vi "GetGrabberPositions.vi"(0 "reference":refnum<class "PackageNode.lvclass">, 5 "error in (no error)":errorcluster) -> (14 "reference out":refnum<class "PackageNode.lvclass">, 15 "GrabberPositions":T2[](array[typedef]) {"y" format="%.2f"; "x" format="%.2f"}, 16 "HotSpots":T1[](array[typedef]) {"HotSpot"."y" format="%.2f"; "HotSpot"."x" format="%.2f"}, 19 "error out":errorcluster)   [LabVIEW 2012, in "PackageNode.lvclass"]
doc: "public Rectangle2D getBounds(Graphics2D g2)"
uses:
  <resource>/Framework/Providers/Open_GDS/UML/PackageNode_class/PackageNode.lvclass
  <resource>/Framework/Providers/Open_GDS/UML/General/Point/Point Point2D.ctl
  <resource>/Framework/Providers/Open_GDS/UML/UMLEditor/UMLEditor_HotSpotData.ctl
  <resource>/Framework/Providers/Open_GDS/UML/AbstractNode_class/AbstractNode.lvclass
  <resource>/Framework/Providers/Open_GDS/UML/UMLEditor/UMLEditor_HotSpotType.ctl
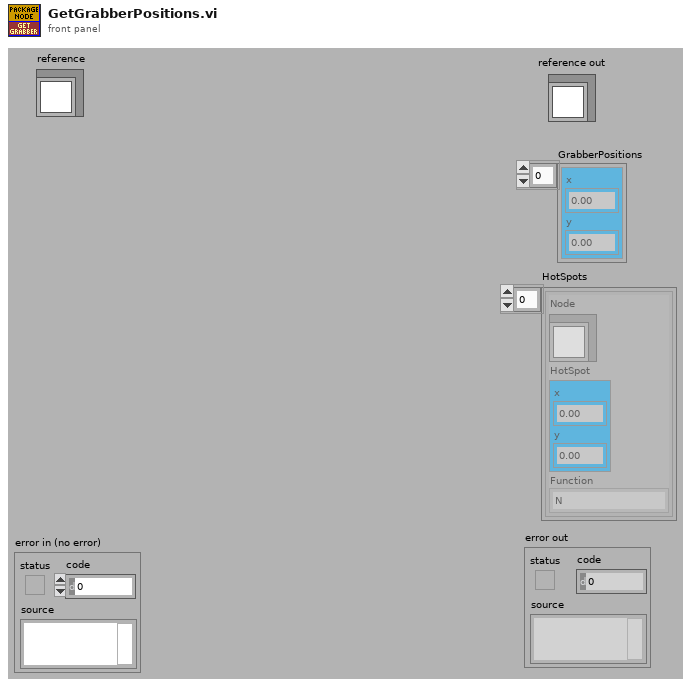
[diagram p1: front panel]
types:
  T1 = typedef "UMLEditor_HotSpotData.ctl" = cluster{"Node":refnum<class "AbstractNode.lvclass">, "HotSpot":T2, "Function":T3}
  T2 = typedef "Point Point2D.ctl" = cluster{"x":dbl, "y":dbl}
  T3 = typedef "UMLEditor_HotSpotType.ctl" = enum16{"N", "NE", "E", "SE", "S", "SW", "W", "NW", "Expand", "Collaps"}
  T4 = typedef "PackageNode.lvclass/ObjectAttributes.ctl" = cluster{"Base class":T5, "name":string, "contents":refnum<class "MultiLineString.lvclass">, "DEFAULT_TOP_WIDTH":i32, "DEFAULT_TOP_HEIGHT":i32, "DEFAULT_WIDTH":i32, "DEFAULT_HEIGHT":i32, "NAME_GAP":i32, "XGAP":i32, "YGAP":i32, "Collapsed":bool, "Note color":u32, "Justification":u16}
  T5 = typedef "RectangularNode.lvclass/ObjectAttributes.ctl" = cluster{"Base class":T6, "bounds":T7}
  T6 = typedef "AbstractNode.lvclass/ObjectAttributes.ctl" = cluster{"parent":refnum<class "AbstractNode.lvclass">, "children":refnum<class "AbstractNode.lvclass">[], "Hidden":bool}
  T7 = typedef "Rectangle Rectangle2D.ctl" = cluster{"x":dbl, "y":dbl, "width":dbl, "height":dbl}
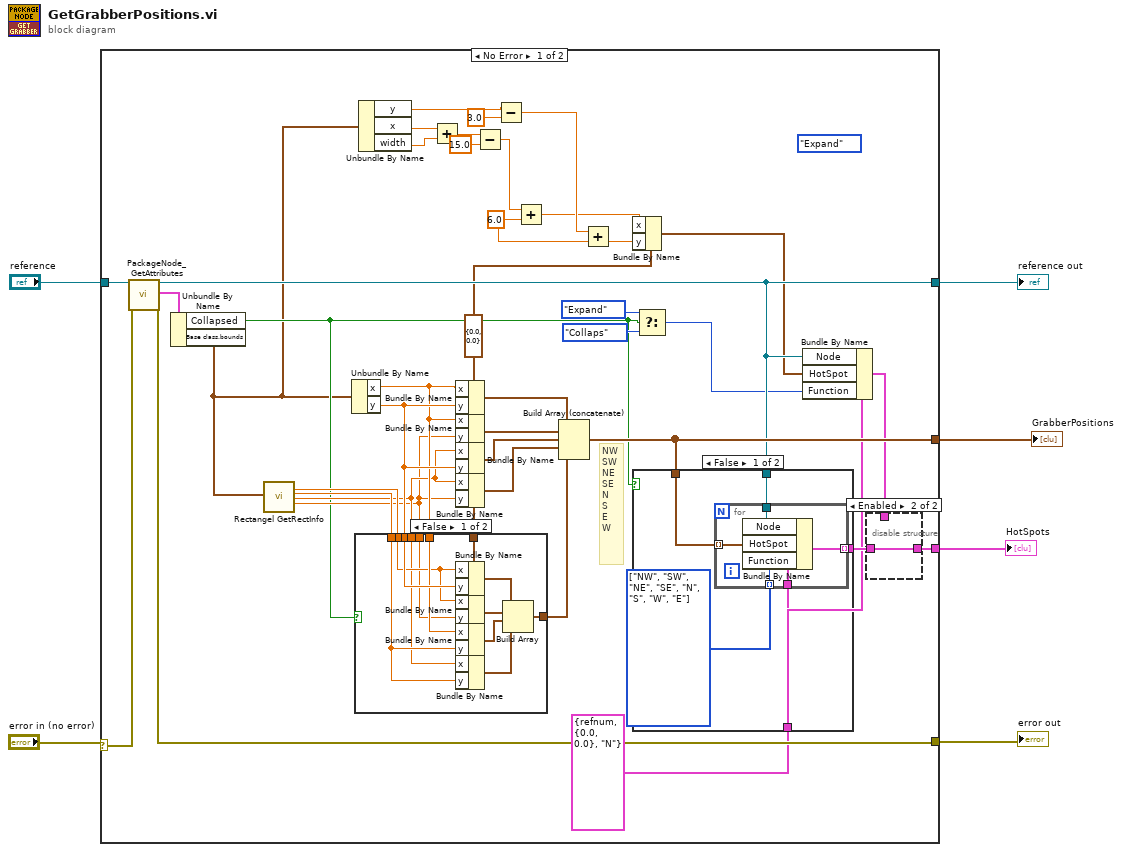
[diagram p0: block diagram]
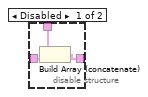
[diagram p4: hidden frame]
diagram:
  n1 = case shown="No Error" "error in (no error)" {
    selector: "error in (no error)" -> [w32 w72]
    tunnel: "reference" -> [w33 w73]
    tunnel: [w31 w72] -> w5
    tunnel: [w25 w73] -> w4
    tunnel: [w34 _] -> w2
    tunnel: [w26 _] -> w1
    frame No Error {
      w27 = T1 {"Node"=refnum, "HotSpot"={"x"=0.0, "y"=0.0}, "Function"=enum."N"} ("ObjectHotSpot")
      (unwired) UMLEditor_HotSpotType."Expand" ("Positions")
      w12 = T2 {"x"=0.0, "y"=0.0} ("point2D")
      w16 = 6.0 ("y")
      # "NW\nSW\nNE\nSE\nN\nS\nE\nW"
      n2 = call <resource>:"PackageNode_GetAttributes.vi"("reference in"=w33, "error in (no error)"=w32) -> ("reference out"=w25:refnum<class "PackageNode.lvclass">, "Attributes"=w30:T4, "error out"=w31:errorcluster)  [unwired: 14 in, 1 out]
      n3 = Unbundle By Name(w30) -> ("Collapsed"=w8:bool, "Base class.bounds"=w7:T7)
      n4 = call <resource>:"Rectangel GetRectInfo.vi"("bounds"=w7) -> ("centerX"=w38:dbl, "centerY"=w37:dbl, "maxX"=w36:dbl, "maxY"=w35:dbl)  [unwired: 1 in, 14 out]
      n5 = Unbundle By Name(w7) -> ("x"=w39:dbl, "y"=w41:dbl)
      n6 = case shown="False" w8 {
        tunnel: w41 -> [w53 _]
        tunnel: [w52 _] -> w40
        tunnel: w39 -> [w51 _]
        tunnel: w38 -> [w50 _]
        tunnel: w37 -> [w49 _]
        tunnel: w36 -> [w48 _]
        tunnel: w35 -> [w47 _]
        tunnel: w12 -> [w46 _]
        frame False {
          n7 = Bundle By Name(cluster=w46, "x"=w50, "y"=w53) -> (w54:T2)
          n8 = Bundle By Name(cluster=w46, "x"=w50, "y"=w47) -> (w55:T2)
          n9 = Bundle By Name(cluster=w46, "x"=w51, "y"=w49) -> (w56:T2)
          n10 = Bundle By Name(cluster=w46, "x"=w48, "y"=w49) -> (w57:T2)
          n11 = Build Array(w54, w55, w56, w57) -> (w52:T2[])
        }
        frame True {
        }
      }
      n12 = Unbundle By Name(w7) -> ("y"=w15:dbl, "x"=w21:dbl, "width"=w20:dbl)
      n13 = Add(x=w21, y=w20) -> (x+y=w19:dbl)
      n14 = Bundle By Name(cluster=w12, "x"=w39, "y"=w41) -> (w45:T2)
      n15 = Bundle By Name(cluster=w12, "x"=w39, "y"=w35) -> (w44:T2)
      n16 = Bundle By Name(cluster=w12, "x"=w36, "y"=w41) -> (w43:T2)
      n17 = Bundle By Name(cluster=w12, "x"=w36, "y"=w35) -> (w42:T2)
      n18 = Subtract(x=w19, y=15.0) -> (x-y=w17:dbl)
      n19 = Subtract(x=w15, y=3.0) -> (x-y=w14:dbl)
      n20 = Add(x=w17, y=w16) -> (x+y=w11:dbl)
      n21 = Build Array (concatenate)(w45, w44, w43, w42, w40) -> (w34:T2[])
      n22 = Add(x=w14, y=w16) -> (x+y=w10:dbl)
      n23 = Bundle By Name(cluster=w12, "x"=w11, "y"=w10) -> (w9:T2)
      n24 = case shown="False" w8 {
        tunnel: w34 -> [w61 _]
        tunnel: [w60 _] -> w29
        tunnel: w27 -> [w59 _]
        tunnel: w25 -> [w58 _]
        frame False {
          w62 = T3[] [enum."NW", enum."SW", enum."NE", enum."SE", enum."N", enum."S", enum."W", enum."E"] items=["N", "NE", "E", "SE", "S", "SW", "W", "NW", "Expand", "Collaps"]
          n25 = for {
            tunnel: w59 -> [w67]
            tunnel: [w66] -> w60 mode=indexing
            tunnel: w62 -> [w65] mode=indexing
            tunnel: w61 -> [w64] mode=indexing
            tunnel: w58 -> [w63]
            n26 = Bundle By Name(cluster=w67, "Node"=w63, "HotSpot"=w64, "Function"=w65) -> (w66:T1)
          }
        }
        frame True {
        }
      }
      n27 = Select(t=UMLEditor_HotSpotType."Expand" ("Positions"), s=w8, f=UMLEditor_HotSpotType."Collaps" ("Positions")) -> (s? t:f=w22:T3)
      n28 = Bundle By Name(cluster=w27, "Node"=w25, "HotSpot"=w9, "Function"=w22) -> (w28:T1)
      n29 = disable-structure shown="Enabled" {
        disable-tunnel: w29 -> [w70 w71]
        disable-tunnel: w28 -> [w69 _]
        disable-tunnel: [w68 w71] -> w26
        frame Disabled {
          n30 = Build Array (concatenate)(w69, w70) -> (w68:T1[])
        }
        frame Enabled {
        }
      }
    }
    frame Error {
    }
  }
  "reference out" <- w4
  "error out" <- w5
  "GrabberPositions" <- w2
  "HotSpots" <- w1
